vi "ParseValue.vi"(8 "error in (no error)":errorcluster, 10 "Index In":i32, 11 "JSON String":string) -> (0 "error out":errorcluster, 2 "Index Out":i32, 3 "JSON Tree":variant)   [LabVIEW 2014, in "i3-json.lvlib"]
doc: "Use this template to build a VI to use as a subVI."
uses:
  i3-json.lvlib
  JSON Types/JSON Type.ctl
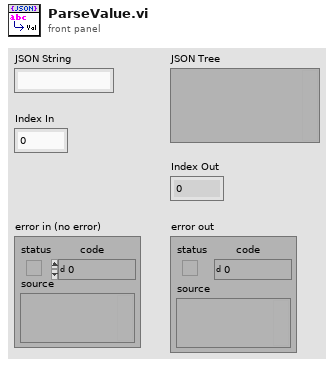
[diagram p1: front panel]
types:
  T1 = typedef "i3-json.lvlib/JSON Type.ctl" = enum8{"JSON Compatible", "JSON Array", "JSON Object", "JSON Null", "Double", "String", "Boolean", "Unknown"}
  T2 = typedef "i3-json.lvlib/Token.ctl" = enum16{"NONE", "CURLY_OPEN", "CURLY_CLOSE", "SQUARED_OPEN", "SQUARED_CLOSE", "COLON", "COMMA", "STRING", "NUMBER", "TRUE", "FALSE", "NULL"}
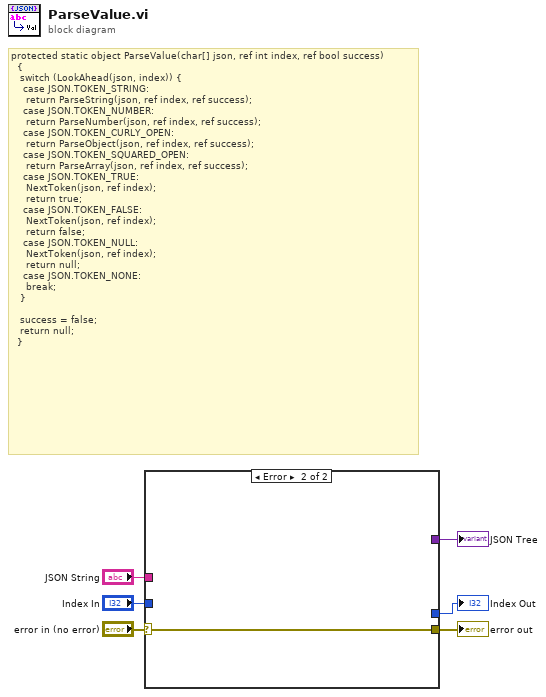
[diagram p0: block diagram]
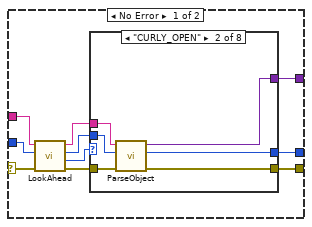
[diagram p2: hidden frame]
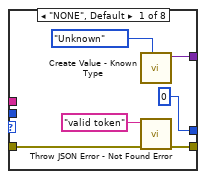
[diagram p3: hidden frame]
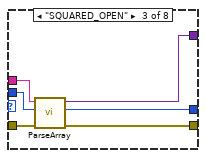
[diagram p4: hidden frame]
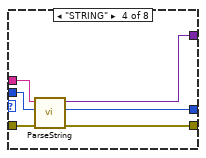
[diagram p5: hidden frame]
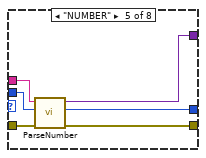
[diagram p6: hidden frame]
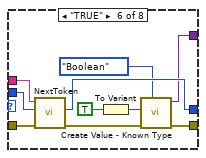
[diagram p7: hidden frame]
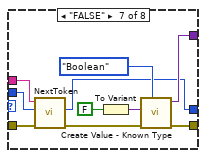
[diagram p8: hidden frame]
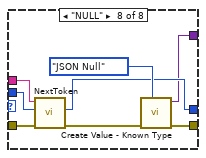
[diagram p9: hidden frame]
diagram:
  # "protected static object ParseValue(char[] json, ref int index, ref bool success)\n\t\t{\n\t\t\tswitch (LookAhead(json, index)) {\n\t\t\t\tcase JSON.TOKEN_STRING:\n\t\t\t\t\treturn ParseString(json, ref index, ref success);\n\t\t\t\tcase JSON.TOKEN_NUMBER:\n\t\t\t\t\treturn ParseNumber(json, ref index, ref success);\n\t\t\t\tcase JSON.TOKEN_CURLY_OPEN:\n\t\t\t\t\treturn ParseObject(json, ref index, ref success);\n\t\t\t\tcase JSON.TOKEN_SQUARED_OPEN:\n\t\t\t\t\treturn ParseArray(json, ref index, ref success);\n\t\t\t\tcase JSON.TOKEN_TRUE:\n\t\t\t\t\tNextToken(json, ref index);\n\t\t\t\t\treturn true;\n\t\t\t\tcase JSON.TOKEN_FALSE:\n\t\t\t\t\tNextToken(json, ref index);\n\t\t\t\t\treturn false;\n\t\t\t\tcase JSON.TOKEN_NULL:\n\t\t\t\t\tNextToken(json, ref index);\n\t\t\t\t\treturn null;\n\t\t\t\tcase JSON.TOKEN_NONE:\n\t\t\t\t\tbreak;\n\t\t\t}\n\n\t\t\tsuccess = false;\n\t\t\treturn null;\n\t\t}"
  n1 = case shown="Error" "error in (no error)" {
    selector: "error in (no error)" -> [w16 w75]
    tunnel: [w14 w75] -> w5
    tunnel: "JSON String" -> [w10 _]
    tunnel: "Index In" -> [w9 _]
    tunnel: [w8 _] -> w2
    tunnel: [w7 _] -> w1
    frame No Error {
      n2 = call "LookAhead.vi"("error in (no error)"=w16, "Index"=w9, "JSON String"=w10) -> ("error out"=w15:errorcluster, "TOKEN"=w13:T2, "Index Passthrough"=w11:i32, "JSON String Passthrough"=w12:string)  [unwired: 4 in]
      n3 = case shown="\"CURLY_OPEN\"" w13 {
        tunnel: w15 -> [w18 w26 w32 w38 w44 w53 w59 w70]
        tunnel: [w17 w25 w31 w37 w43 w52 w61 w68] -> w14
        tunnel: [w21 w23 w29 w35 w41 w51 w62 w67] -> w8
        tunnel: w12 -> [_ w27 w34 w40 w46 w56 w57 w72]
        tunnel: w11 -> [_ w28 w33 w39 w45 w55 w58 w71]
        tunnel: [0 ("Index Out") w24 w30 w36 w42 w54 w60 w69] -> w7
        frame "NONE", Default {
          n4 = call "Create Value - Known Type.vi"("JSON Type"=JSON_Type."Unknown") -> ("JSON Tree"=w21:variant)  [unwired: 9 in, 1 out]
          n5 = call "Throw JSON Error - Not Found Error.vi"("error in (no error)"=w18, "item type"="valid token") -> ("error out"=w17:errorcluster)  [unwired: 9 in]
        }
        frame "CURLY_OPEN" {
          n6 = call "ParseObject.vi"("error in (no error)"=w26, "Index In"=w28, "JSON String"=w27) -> ("error out"=w25:errorcluster, "Index Out"=w24:i32, "JSON Tree"=w23:variant)  [unwired: 6 in]
        }
        frame "SQUARED_OPEN" {
          n7 = call "ParseArray.vi"("error in (no error)"=w32, "Index In"=w33, "JSON String"=w34) -> ("error out"=w31:errorcluster, "Index Out"=w30:i32, "JSON Tree"=w29:variant)  [unwired: 6 in]
        }
        frame "STRING" {
          n8 = call "ParseString.vi"("error in (no error)"=w38, "Index In"=w39, "JSON String"=w40) -> ("error out"=w37:errorcluster, "Index Out"=w36:i32, "JSON Tree"=w35:variant)  [unwired: 5 in, 1 out]
        }
        frame "NUMBER" {
          n9 = call "ParseNumber.vi"("error in (no error)"=w44, "Index In"=w45, "JSON String"=w46) -> ("error out"=w43:errorcluster, "Index Out"=w42:i32, "JSON Tree"=w41:variant)  [unwired: 6 in]
        }
        frame "TRUE" {
          n10 = call "NextToken.vi"("error in (no error)"=w53, "Index In"=w55, "JSON String"=w56) -> ("error out"=w50:errorcluster, "Index Out"=w54:i32)  [unwired: 4 in, 2 out]
          n11 = To Variant(anything=TRUE) -> (Variant=w47:variant)
          n12 = call "Create Value - Known Type.vi"("JSON Type"=JSON_Type."Boolean", "error in (no error)"=w50, "Value"=w47) -> ("error out"=w52:errorcluster, "JSON Tree"=w51:variant)  [unwired: 7 in]
        }
        frame "FALSE" {
          n13 = call "NextToken.vi"("error in (no error)"=w59, "Index In"=w58, "JSON String"=w57) -> ("error out"=w66:errorcluster, "Index Out"=w60:i32)  [unwired: 4 in, 2 out]
          n14 = To Variant(anything=FALSE) -> (Variant=w63:variant)
          n15 = call "Create Value - Known Type.vi"("JSON Type"=JSON_Type."Boolean", "error in (no error)"=w66, "Value"=w63) -> ("error out"=w61:errorcluster, "JSON Tree"=w62:variant)  [unwired: 7 in]
        }
        frame "NULL" {
          n16 = call "NextToken.vi"("error in (no error)"=w70, "Index In"=w71, "JSON String"=w72) -> ("error out"=w74:errorcluster, "Index Out"=w69:i32)  [unwired: 4 in, 2 out]
          n17 = call "Create Value - Known Type.vi"("JSON Type"=JSON_Type."JSON Null", "error in (no error)"=w74) -> ("error out"=w68:errorcluster, "JSON Tree"=w67:variant)  [unwired: 8 in]
        }
      }
    }
    frame Error {
    }
  }
  "error out" <- w5
  "JSON Tree" <- w2
  "Index Out" <- w1
